vi "Tokenize Tag.vi"(8 "Error In":errorcluster, 11 "Lexer In":refnum<class "Lexer.lvclass">) -> (0 "Error Out":errorcluster, 3 "Lexer Out":refnum<class "Lexer.lvclass">)   [LabVIEW 2018, in "Toolkit.lvlib" / "Lexer.lvclass"]
uses:
  Lexer.lvclass
  Lexer.lvclass/Lexer.ctl
  Tokens/EscapedVariable/EscapedVariable.lvclass
  D:/Users/cfield/Code/Field R&D Services/Labstache/src/Toolkit/Low-Level/Tokens/Token/Token.lvclass
  Tokens/Comment/Comment.lvclass
  Tokens/UnescapedVariable/UnescapedVariable.lvclass
  Tokens/BeginSection/BeginSection.lvclass
  Tokens/InvertedSection/InvertedSection.lvclass
  Tokens/EndSection/EndSection.lvclass
  Tokens/Partial/Partial.lvclass
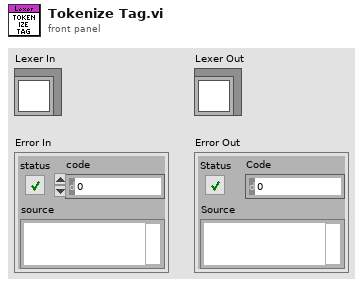
[diagram p1: front panel]
types:
  T1 = typedef "Toolkit.lvlib/Delimiters.ctl" = cluster{"Close":string, "Open":string}
  T2 = typedef "Toolkit.lvlib/Lexer.lvclass/Tag Types.ctl" = enum16{"Escaped Variable", "{} Unescaped Variable", "& Unescaped Variable", "Begin Section", "Inverted Section", "End Section", "Comment", "Partial", "Set Delimiter"}
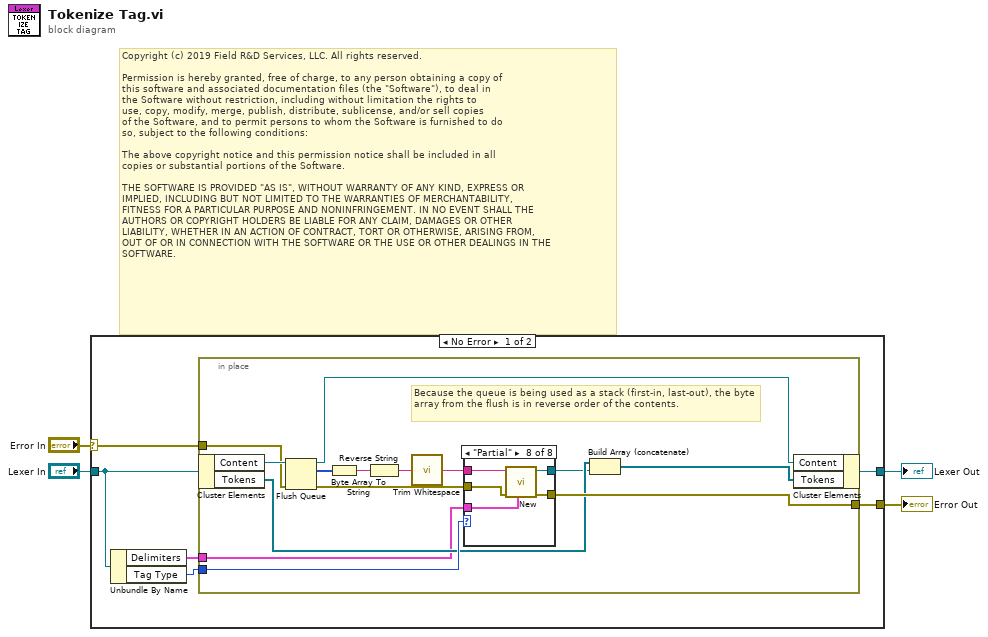
[diagram p0: block diagram]
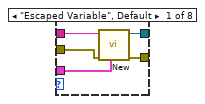
[diagram p2: hidden frame]
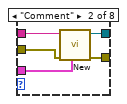
[diagram p3: hidden frame]
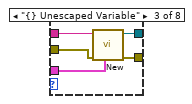
[diagram p4: hidden frame]
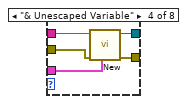
[diagram p5: hidden frame]
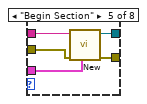
[diagram p6: hidden frame]
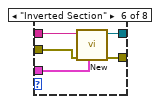
[diagram p7: hidden frame]
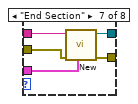
[diagram p8: hidden frame]
diagram:
  # "Copyright (c) 2019 Field R&D Services, LLC. All rights reserved.\n\nPermission is hereby granted, free of charge, to any person obtaining a copy of\nthis software and associated documentation files (the \"Software\"), to deal in\nthe Software without restriction, including without limitation the rights to\nuse, copy, modify, merge, publish, distribute, sublicense, and/or sell copies\nof the Software, and to permit persons to whom the Software is furnished to do\nso, subject to the following conditions:\n\nThe above copyright notice and this permission notice shall be included in all\ncopies or substantial portions of the Software.\n\nTHE SOFTWARE IS PROVIDED \"AS IS\", WITHOUT WARRANTY OF ANY KIND, EXPRESS OR\nIMPLIED, INCLUDING BUT NOT LIMITED TO THE WARRANTIES OF MERCHANTABILITY,\nFITNESS FOR A PARTICULAR PURPOSE AND NONINFRINGEMENT. IN NO EVENT SHALL THE\nAUTHORS OR COPYRIGHT HOLDERS BE LIABLE FOR ANY CLAIM, DAMAGES OR OTHER\nLIABILITY, WHETHER IN AN ACTION OF CONTRACT, TORT OR OTHERWISE, ARISING FROM,\nOUT OF OR IN CONNECTION WITH THE SOFTWARE OR THE USE OR OTHER DEALINGS IN THE\nSOFTWARE."
  n1 = case shown="No Error" "Error In" {
    selector: "Error In" -> [w8 w65]
    tunnel: [w10 w65] -> w4
    tunnel: [w9 w66] -> w3
    tunnel: "Lexer In" -> [w7 w66]
    frame No Error {
      n2 = Unbundle By Name(w7) -> ("Delimiters"=w5:T1, "Tag Type"=w6:T2)
      n3 = in-place {
        in-place-border: [w17] -> w10
        in-place-border: w8 -> [w21]
        in-place-border: w6 -> [w15]
        in-place-border: w5 -> [w11]
        # "Because the queue is being used as a stack (first-in, last-out), the byte array from the flush is in reverse order of the contents."
        n4 = in-place-cluster #1(w7) -> ("Content"=w24:refnum<queue>, "Tokens"=w14:refnum<class "Token.lvclass">[])
        n5 = Flush Queue(queue=w24, error in (no error)=w21) -> (queue out=w23:refnum<queue>, remaining elements=w22:u8[], error out=w18:errorcluster)
        n6 = Byte Array To String(unsigned byte array=w22) -> (string=w20:string)
        n7 = Reverse String(1:w20) -> (0:w19:string)
        n8 = call <vilib>:"Trim Whitespace.vi"("string"=w19) -> ("trimmed string"=w16:string)  [unwired: 1 in]
        n9 = case shown="\"Partial\"" w15 {
          tunnel: w18 -> [w29 w32 w38 w43 w48 w53 w58 w63]
          tunnel: [w28 w31 w37 w42 w47 w52 w57 w62] -> w17
          tunnel: w16 -> [w27 w34 w39 w44 w49 w54 w59 w64]
          tunnel: [w26 w33 w36 w41 w46 w51 w56 w61] -> w13
          tunnel: w11 -> [w25 w30 w35 w40 w45 w50 w55 w60]
          frame "Escaped Variable", Default {
            n10 = call "New.vi"("Delimiters"=w25, "Error In"=w29, "Key"=w27) -> ("Error Out"=w28:errorcluster, "Escaped Variable"=w26:refnum<class "EscapedVariable.lvclass">)  [unwired: 7 in]
          }
          frame "Comment" {
            n11 = call "New.vi"("Delimiters"=w30, "Error In"=w32, "Content"=w34) -> ("Error Out"=w31:errorcluster, "Comment"=w33:refnum<class "Comment.lvclass">)  [unwired: 7 in]
          }
          frame "{} Unescaped Variable" {
            n12 = call "New.vi"("Delimiters"=w35, "Error In"=w38, "Key"=w39) -> ("Error Out"=w37:errorcluster, "Unescaped Variable"=w36:refnum<class "UnescapedVariable.lvclass">)  [unwired: 7 in]
          }
          frame "& Unescaped Variable" {
            n13 = call "New.vi"("Delimiters"=w40, "Error In"=w43, "Key"=w44) -> ("Error Out"=w42:errorcluster, "Unescaped Variable"=w41:refnum<class "UnescapedVariable.lvclass">)  [unwired: 7 in]
          }
          frame "Begin Section" {
            n14 = call "New.vi"("Delimiters"=w45, "Error In"=w48, "Key"=w49) -> ("Error Out"=w47:errorcluster, "Begin Section"=w46:refnum<class "BeginSection.lvclass">)  [unwired: 7 in]
          }
          frame "Inverted Section" {
            n15 = call "New.vi"("Delimiters"=w50, "Error In"=w53, "Key"=w54) -> ("Error Out"=w52:errorcluster, "Inverted Section"=w51:refnum<class "InvertedSection.lvclass">)  [unwired: 7 in]
          }
          frame "End Section" {
            n16 = call "New.vi"("Delimiters"=w55, "Error In"=w58, "Key"=w59) -> ("Error Out"=w57:errorcluster, "End Section"=w56:refnum<class "EndSection.lvclass">)  [unwired: 7 in]
          }
          frame "Partial" {
            n17 = call "New.vi"("Delimiters"=w60, "Error In"=w63, "Key"=w64) -> ("Error Out"=w62:errorcluster, "Partial"=w61:refnum<class "Partial.lvclass">)  [unwired: 7 in]
          }
        }
        n18 = Build Array (concatenate)(w14, w13) -> (w12:refnum<class "Token.lvclass">[])
        n19 = in-place-cluster #1("Content"=w23, "Tokens"=w12) -> (w9:refnum<class "Lexer.lvclass">)
      }
    }
    frame Error {
    }
  }
  "Error Out" <- w4
  "Lexer Out" <- w3
